vi "Exercise introduction.vi"(5 "Exercise Execution Mode":T1, 6 "Numero USP":dbl format="%#.13f", 7 "Exercise Number":T6, 8 "error in":errorcluster, 9 "Waveform In":waveform(dbl), 10 "Array":bool[](array[boolean]), 11 "Exercise Folder Path":path) -> (0 "error out":errorcluster, 1 "Waveform Out":waveform(dbl), 2 "Done":dbl, 3 "path":path)   [LabVIEW 2014]
uses:
  Ctls/t2q1.ctl
  Ctls/t2q2.ctl
  Ctls/ExerciseNumeration.ctl
  Ctls/ExerciseState.ctl
  Ctls/teval.ctl
  <vilib>/Utility/miscctls.llb/LVPointTypeDef.ctl
  Ctls/radiobutton010.ctl
panel:
  out "Exercise Tab":T2(tab)
  in  "Close 3":bool
  in  "TEVAL":T3 caption="Perguntas"
  in  "Close":bool
  in  "T2E1":T4 caption="Perguntas:"
  in  "Help? 2":bool
  out "Ex1 Graph Overview":waveform(dbl)(graph)
  in  "T2E2":T5={"Vmax (V)"=0.0, "Vmin (V)"=0.0, "Taxa de Aquisição (Hz)"=0.0, "Resolução (bits)"=0.0, "Amplificação (V/V)"=1.0, "V+(V)"=0.0, "V- (V)"=0.0, "LSB (V)"=0.0}
  in  "Close 2":bool
  in  "Help? 3":bool
  # "PSI3214\nLaboratório de Instrumentação Elétrica"
  # "Avaliação do Tutorial"
  # "Ao longo do tutorial foram utilizados materiais em PDF para referência do aluno, materiais em vídeo para acompanhamento mais dinâmico. Neste questionário serão avaliados alguns parâmetros quantitativos a fim de se melhorar a qualidade dos tutoriais fornecidos ao longo dos anos. É importante deixar claro que não será pedida nenhuma informação que possa identificar o aluno, de modo a preservar a privacidade de cada um."
  # "AA.1) Em relação ao Material Escrito disponibilizado em PDF, avalie:"
  # "Neste tutorial você foi apresentado a diversos conceitos sobre instrumentação elétrica e programação em LabVIEW. Em relação ao tamanho e à quantidade de conteúdo apresentado, você qualifica o tutorial como:"
  # "Pouco extenso\nPouco conteúdo"
  # "Pouco Extenso\nConteúdo adequado"
  # "Muito Extenso\nConteúdo adequado"
  # "Muito extenso\nPouco conteúdo"
  # "A realização dos tutoriais é importante para ter uma experiência completa do Laboratório de Instrumentação Elétrica. No entanto, é necessário um balanço entre as aulas teórias, experimentos e o exercícios em LabVIEW. Estime o tempo utilizado para a realização deste tutorial:"
  # "00h30-"
  # "00h30"
  # "01h00"
  # "01h30"
  # "02h00"
  # "02h30"
  # "03h00"
  # "03h30"
  # "04h00"
  # "04h00+"
  # "Este tutorial foi elaborado para ser realizado em conjunto com as disciplinas oferecidas no 4º semestre do curso de Engenharia Elétrica. Com relação aos conceitos abordados neste tutorial, indique, na sua opinião, que parcela do conteúdo foi apresentada adequadamente:"
  # "Nenhuma"
  # "Poucos"
  # "Maioria"
  # "Todos"
  # "Dada a quantidade de conceitos novos apresentados ao longo do tutorial, estime quantas leituras, em média, foram utilizadas para a compreensão de um tópico:"
  # "4 vezes +"
  # "3 vezes"
  # "2 vezes"
  # "1 vez"
  # "Apesar do tutorial apresentar novos conteúdos de programação, dentre outros conteúdos, sua proposta é de complementar as aulas teóricas e práticas de laboratório. Na sua opinião, estime como este tutorial auxiliou na compreensão dos assunto tratados na disciplina:"
  # "Dificultou\nmuito"
  # "Dificultou\npouco"
  # "Auxiliou\npouco"
  # "Auxiliou\nmuito"
  # "A instrumentação elétrica apresenta uma vasta gama de problemas de aquisição e processamento de dados. Para compreender melhor como aplicar os conceitos abordados na disciplina, neste tutorial foram apresentados alguns exemplos de problemas de instrumentação na forma de exercícios. Com relação aos problemas apresentados, indique como os exercícios propostos o auxiliaram em sua resolução:"
  # "Exercício não \najudou em nada"
  # "Exercício pouco \najudou na resolução"
  # "Exercício ajudou\nparcialmente na resolução"
  # "Exercício ajudou \nbastante na resolução"
  # "Diversos conceitos sobre programação em LabVIEW foram apresentados no tutorial. Tais ferramentas foram apresentadas com a intenção de ensiná-los como e quando utilizá-las. Estime o seu aprendizado a respeito de como utilizar tais ferramentas de programação e para qual finalidade aplicá-las:"
  # "Não sei como utilizar, \ne não sei sua finalidade"
  # "Sei como utilizar, mas \nnão sei sua finalidade"
  # "Não sei como utilizar, \nmas sei sua finalidade"
  # "Sei como utilizar, \ne sei sua finalidade"
  # "Indique como este tutorial colaborou na compreensão de assuntos abordados por outras disciplinas:"
  # "Nada"
  # "Pouco"
  # "Parcialmente"
  # "Muito"
  # "Indique seu conhecimento prévio a respeito do ambiente de programação em LabVIEW ante de realizar esse tutorial:"
  # "Não sabia o \nque era LabVIEW"
  # "Já tinha ouvido falar, mas \nnunca programei LabVIEW"
  # "Já programei LabVIEW\nalgumas vezes"
  # "Utilizo LabVIEW com\nalguma regularidade"
  # "Dada a resposta do item anterior, indique como classificaria seu aprendizado do conteúdo apresentado:"
  # "Todo o conteúdo\napresentado"
  # "Nada"
  # "Pouco"
  # "Parcialmente"
  # "PSI3214\nLaboratório de Instrumentação Elétrica"
  # "Exercício 2.1"
  # "Vimos ao longo do tutorial 2 que um sistema de aquisição possui como principal componente o ADC, Conversor Analógico Digital ou (Analog to Digital Converter). Para definição dos parâmentros que definem o ADC, tais como sua taxa de aquisição, fundo de escala e sua resolução, é necessário primeiro uma analise do sinal de entrada. Neste primeiro exercício iremos construir um projeto ingênuo de um ADC, desconsiderando algumas sutilezas presentes em sistemas de aquisição."
  # "Uma empresa de motores elétricos quer avaliar qual a precisão da construção de seus motores. Idealmente, os motores possuem rotação de 12000 RPM, contudo, defeitos na construção do eixo principal podem afetar a rotação. Como engenheiro de teste desta empresa à você foi encarregada a tarefa de construção de um sistema de aquisição para realizar tal avaliação. \n\nComo o sistema deve se móvel, você optou pela construção de um sensor de rotação ótico (figura ao lado). A cada rotação completa do eixo central do motor uma fita branca passa na frente do refletor IR, produzindo um pulso que será identificado pelo sistema de conversão AD."
  # "Utilize o sinal gerado no VI do exercicio para responder as perguntas abaixo:"
  # "Para fechar a tela do enunciado, pressione o botão \"Close Form\""
  # "A) Analise o sinal adquirido pelo ADC (em azul) e indique as características à seguir:"
  # "B) Sabe-se que o ADC utilizado para a aquisição inicial é de 10 bits e possui um LSB de aproximadamente 23,43mV. Indique o valor do fundo de escala:"
  # "C) Caso fosse requisitado que o ADC fosse sensível a variações do sinal de no mínimo 0,50mV. Indique os valores de,"
  # "PSI3214\nLaboratório de Instrumentação Elétrica"
  # "Exercício 2.2"
  # "Até o presente momento foi realizada uma apresentação ingênua do problema de aquisição de dados, na qual um conversor AD pode realizar aquisições de dados sem a introdução de erros ou ruídos no sinal qualquer que seja sua tensão de alimentação. Contudo, como discutido no tutorial, não é recomendado que a tensão de alimentação de um conversor seja pequena. Dados os circuitos integrados disponíveis no mercado, tensões de 5V são algumas das mais comuns para aplicações ordinárias."
  # "Como todos os sistemas que operam no mundo real, sempre serão introduzidos erros no sinal. É também trabalho do engenheiro identificar essas fontes de erros e buscar minimizar seus efeitos na análise final. Para o caso específico dos Conversores AD, são introduzidos erros proporcionais àqueles presentes na alimentação do ADC, bem como erros introduzidos por indutâncias e capacitâncias parasitárias. Quando  a tensão de alimentação é muito baixa, a proporção entre os erros introduzidos e o sinal de interesse aumenta, algo indesejado, especialmente para o caso de sinais de baixa amplitude. Caso utilizemos um conversor AD em conjunto com um amplificador, podemos aumentar os níveis do sinal, efetivamente diminuindo a proporção entre erro introduzido e o sinal, como mostra a figura abaixo."
  # "Um dos temas em Engenharia que tem maior adesão da mídia é o de Cidades Inteligentes e a sua construção por meio de sistemas embarcados, capazes de realizar aquisição de dados, processamento e a comunicação desses dados para outros sistemas. Contudo, a ideia de se colocar sensores em uma cidade afim de se monitorar condições como tráfego, níveis de ruído, dentre outros parâmetros não é uma ideia nova. No final dos anos 90 nos EUA, com o aumento dos índices de criminalidade em cidades grandes foram implementados os primeiros projetos de identificação de dispáro de tiros em algumas das principais vias das maiores cidades. Apesar de a classificassão do sinal como sendo de uma arma de fogo ou de uma batida de carro ser um assunto complexo, o sistema de aquisição de dados é, de certo modo, simples. \n    Neste exercício vamos utilizar o diagrama de blocos descrito anteriormente como a topologia de nosso projeto. Como definido acima, iremos fazer uso de um aplificador antes do processo de conversão AD.\n    Utilize o sinal gerado no VI principal para realizar as medições pertinentes:"
  # "A) Descreva o sinal a ser adquirido (em vermelho), indicando:"
  # "- Níveis de Tensão Globais Máximo e Mínimo:"
  # "Na modelagem sonora de uma arma de fogo, sugere-se que para maioria das armas comercializadas estamos interessados em sinais de até 2kHz, sendo assim:"
  # "B) Dado que 20x a Frequência de Nyquist é um valor utilizado em engenharia como mais do que \nadequado para o processo de aquisição de dados, selecione qual a taxa de aquisição mínima mais \naceitável para o conversor AD:"
  # "C) Dado que a tensão de fundo de escala do conversor é de 10V e que desejamos utilzar ao máximo os endereços binários com informação util: Qual a amplificação que deverá ser dada ao sinal (em vermelho)? Dado que o sinal é simétrico, quais as tensões de alimentação do conversor AD para que tenha a tensão de fundo de escala necessária?"
  # "Como etapa final do projeto, queremos que quaisquer variações de sinal menores ou da ordem de 1mV sejam detectadas pelo conversor, deste modo:"
  # "D) Selecione qual a resolução mínima para que essa especificação seja cumprida e qual o LSB resultante desta configuração, considerando a tensão do fundo de escala dada no item C."
  # "Para fechar a tela do enunciado, pressione o botão \"Close Form\""
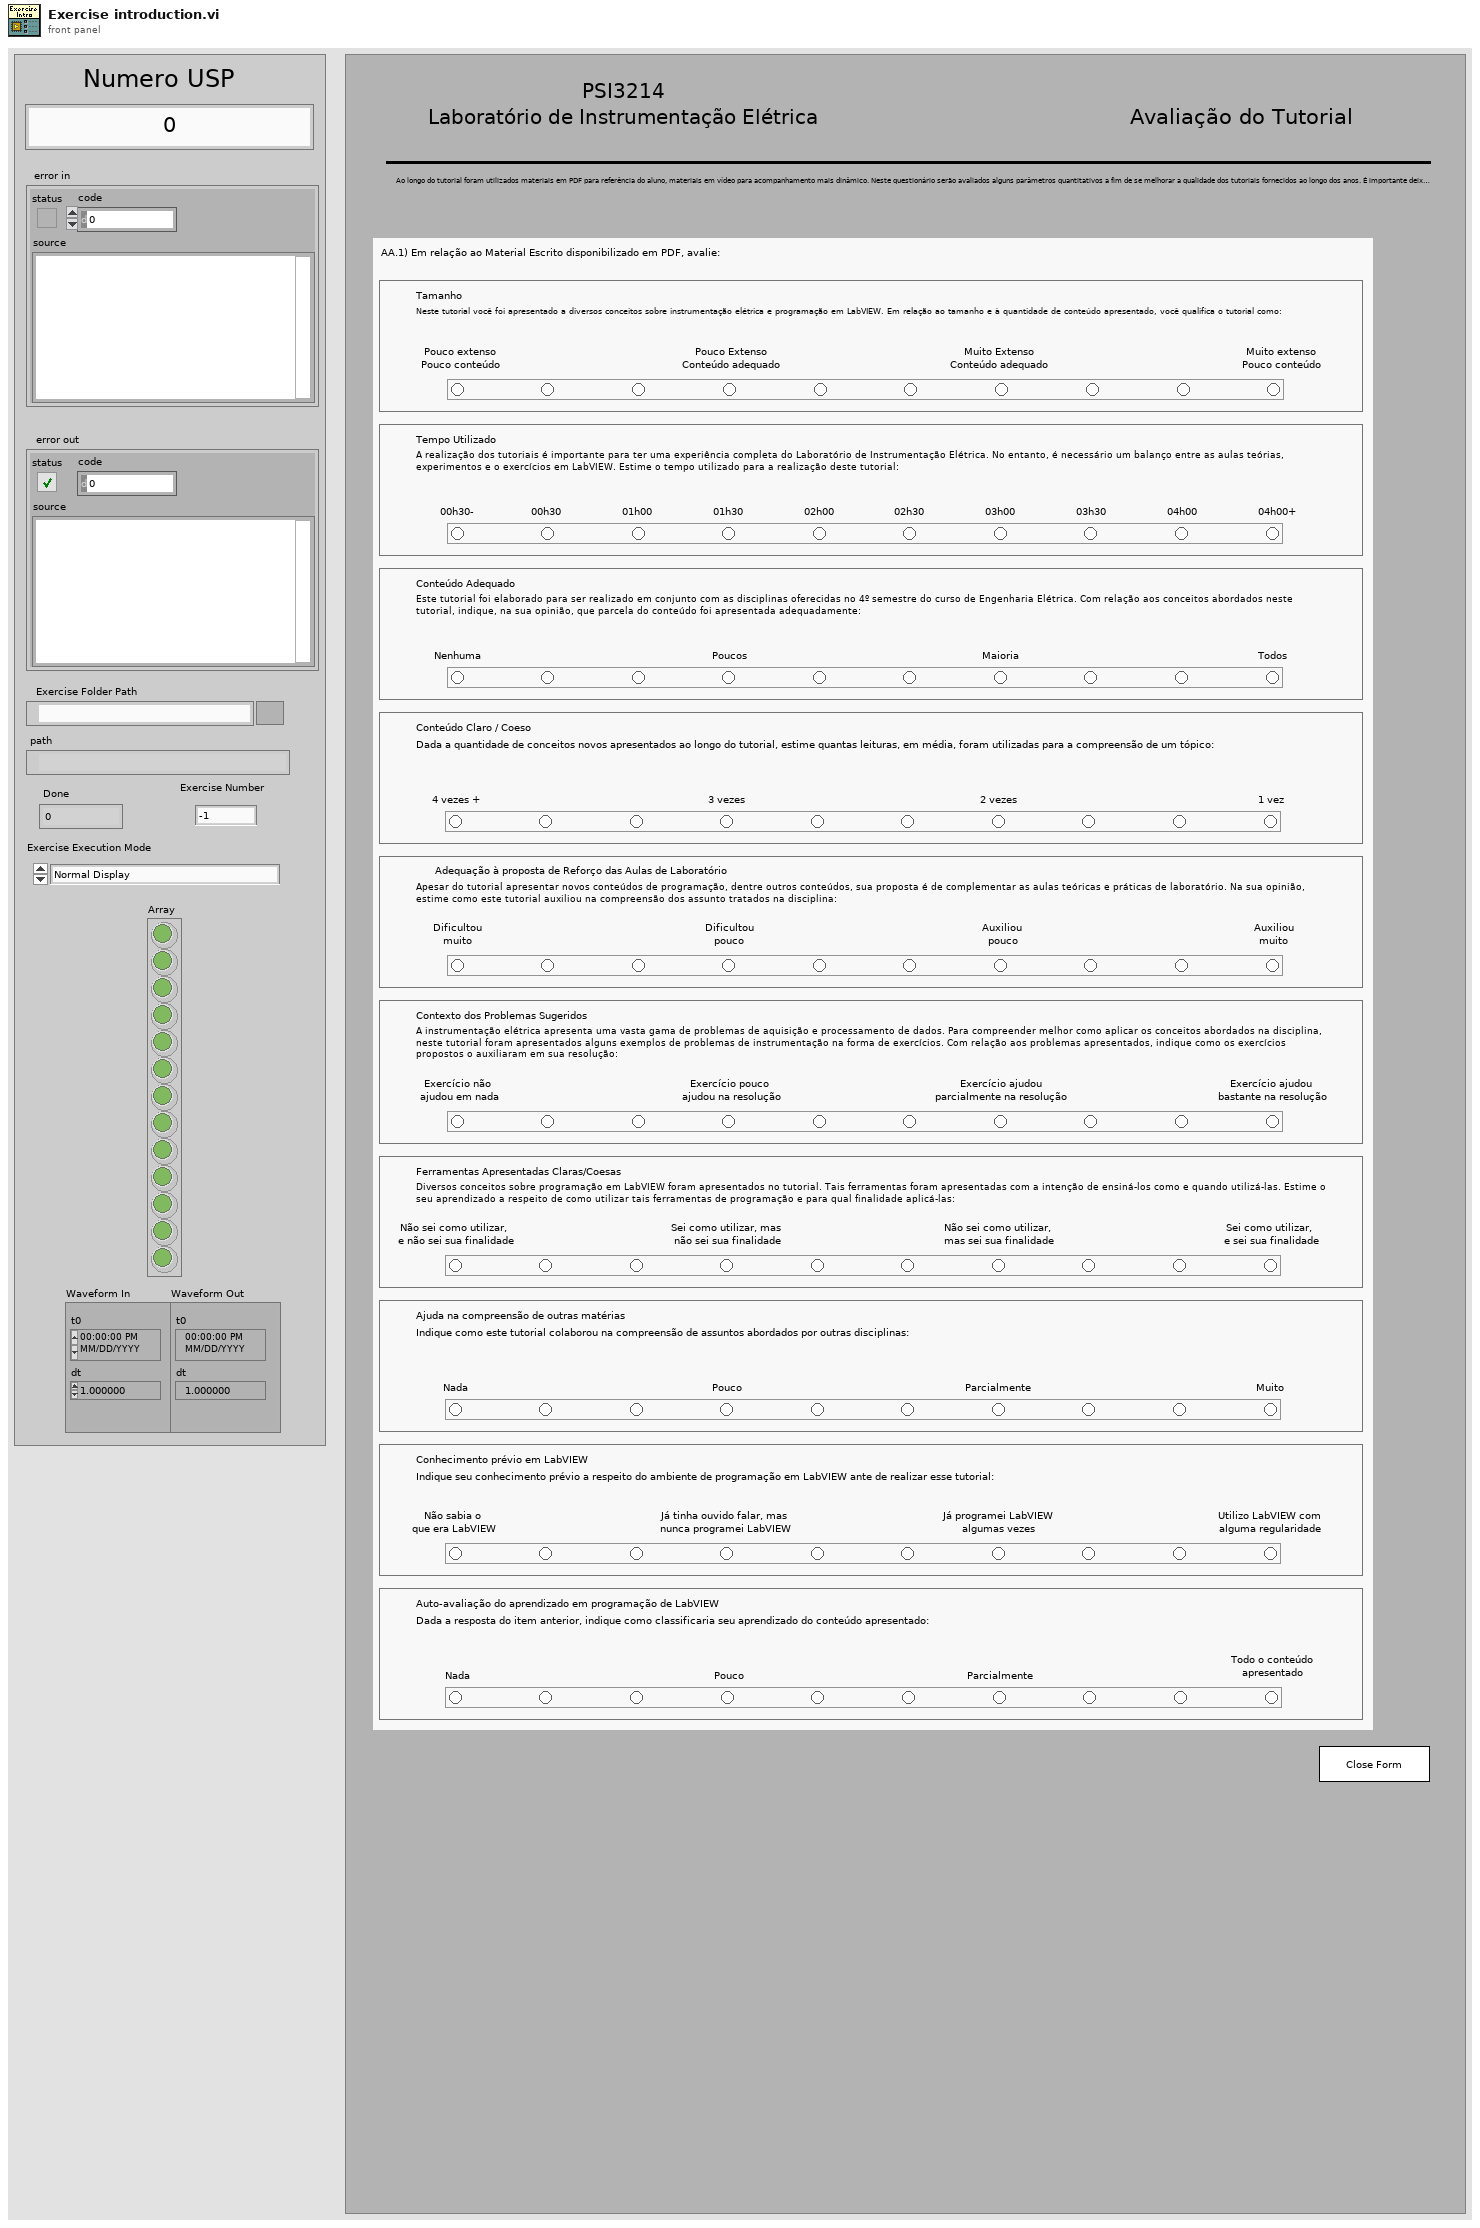
[diagram p1: front panel]
types:
  T1 = typedef "ExerciseState.ctl" = enum16{"Normal Display", "Answer Highligh"}
  T2 = enum32{"Tutorial Evaluation", "Exercicio 1", "Exercicio 2", "Exercício 3", "Exercício 4", "Exercício 5"}
  T3 = typedef "teval.ctl" = cluster{"Tamanho":enum32{"No Selection", "2", "1", "3", "4", "5", "6", "7", "8", "9", "10"}, "Tempo Utilizado":enum32{"No Selection", "2", "1", "3", "4", "5", "6", "7", "8", "9", "10"}, "Conteúdo Adequado":enum32{"No Selection", "2", "1", "3", "4", "5", "6", "7", "8", "9", "10"}, "Conteúdo Claro / Coeso":enum32{"No Selection", "2", "1", "3", "4", "5", "6", "7", "8", "9", "10"}, "Adequação à proposta de Reforço das Aulas de Laboratório e de Ensino de LabVIEW":enum32{"No Selection", "2", "1", "3", "4", "5", "6", "7", "8", "9", "10"}, "Contexto dos Problemas Sugeridos":enum32{"No Selection", "2", "1", "3", "4", "5", "6", "7", "8", "9", "10"}, "Contexto das Ferramentas Apresentadas":enum32{"No Selection", "2", "1", "3", "4", "5", "6", "7", "8", "9", "10"}, "Ajuda na compreensão de outras matérias":enum32{"No Selection", "2", "1", "3", "4", "5", "6", "7", "8", "9", "10"}, "compreensão de programação em LabVIEW":enum32{"No Selection", "2", "1", "3", "4", "5", "6", "7", "8", "9", "10"}, "compreensão da teoria apresentada":enum32{"No Selection", "2", "1", "3", "4", "5", "6", "7", "8", "9", "10"}}
  T4 = typedef "t2q1.ctl" = cluster{"Vmax (V)":dbl, "Vmin (V)":dbl, "Período (s)":dbl, "Fundo de Escala (V)":dbl, "Frequência de \nAmostragem \n[Hz]":dbl, "LSB (V)":dbl, "Resolução (bits)":dbl}
  T5 = typedef "t2q2.ctl" = cluster{"Vmax (V)":dbl, "Vmin (V)":dbl, "Taxa de Aquisição (Hz)":dbl, "Resolução (bits)":dbl, "Amplificação (V/V)":dbl, "V+(V)":dbl, "V- (V)":dbl, "LSB (V)":dbl}
  T6 = typedef "ExerciseNumeration.ctl" = enum16{"-1", "0", "1", "2", "3", "4", "5", "6", "7", "8", "9", "10"}
  T7 = typedef "LVPointTypeDef.ctl" = cluster{"Horizontal":i16, "Vertical":i16}
  T8 = enum16{"Always On", "Always Off", "Off While Running"}
  T9 = enum16{"open", "replace", "create", "open or create", "replace or create", "replace or create with confirmation"}
  T10 = typedef "radiobutton010.ctl" = enum32{"No Selection", "2", "1", "3", "4", "5", "6", "7", "8", "9", "10"}
  T11 = enum32{"No Selection", "2", "1", "3", "4", "5", "6", "7", "8", "9", "10"}
  T12 = enum32{"No Selection", "2", "1", "3", "4", "5", "6", "7", "8", "9", "10"}[]
  T13 = typedef "imagedata.ctl" = cluster{"image type":i32, "image depth":i32, "image":u8[], "mask":u8[], "colors":u32[], "Rectangle":cluster{"left":i16, "top":i16, "right":i16, "bottom":i16}}
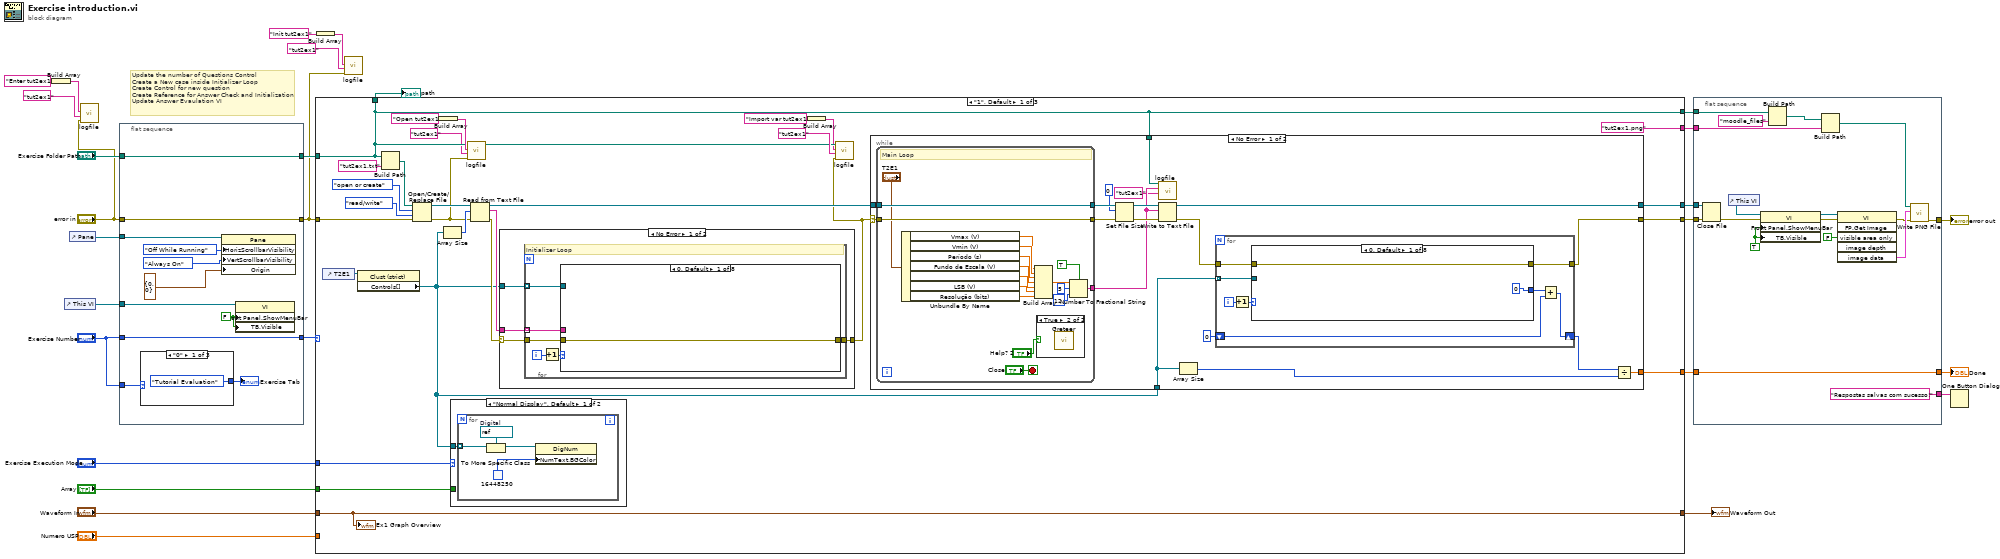
[diagram p0: block diagram]
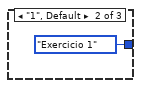
[diagram p2: hidden frame]
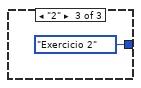
[diagram p3: hidden frame]
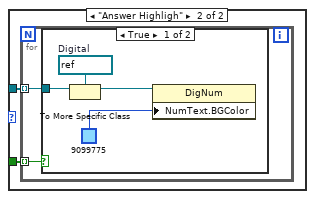
[diagram p4: hidden frame]
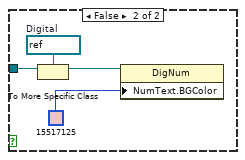
[diagram p5: hidden frame]
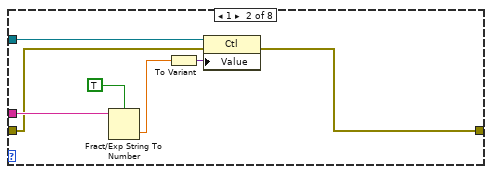
[diagram p6: hidden frame]
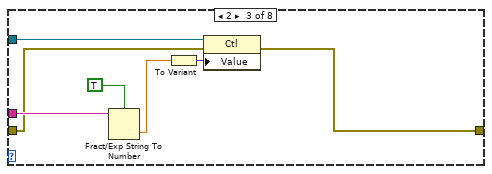
[diagram p7: hidden frame]
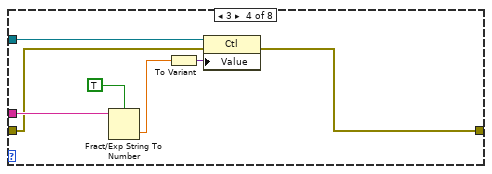
[diagram p8: hidden frame]
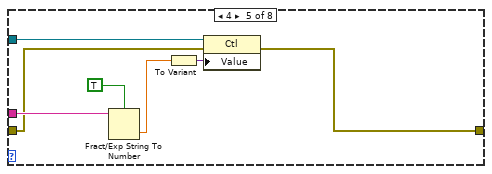
[diagram p9: hidden frame]
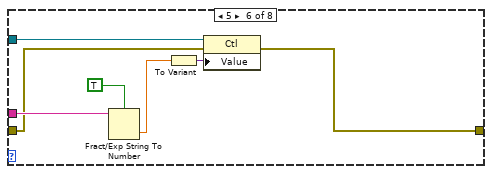
[diagram p10: hidden frame]
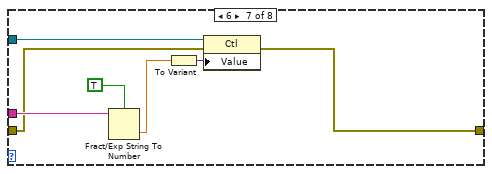
[diagram p11: hidden frame]
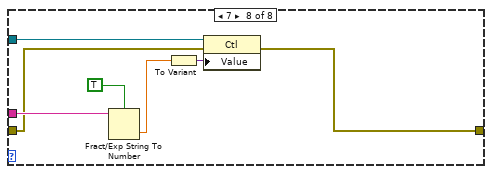
[diagram p12: hidden frame]
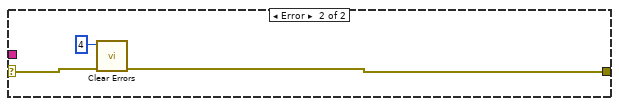
[diagram p13: hidden frame]
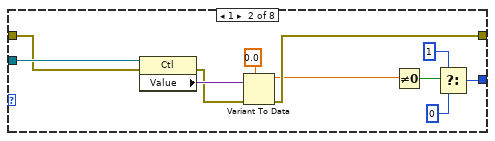
[diagram p14: hidden frame]
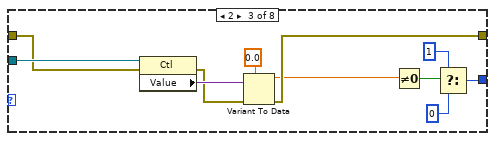
[diagram p15: hidden frame]
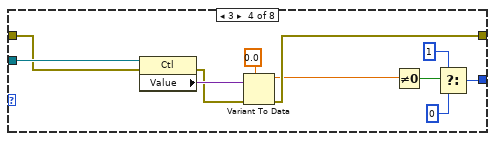
[diagram p16: hidden frame]
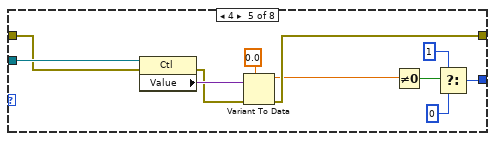
[diagram p17: hidden frame]
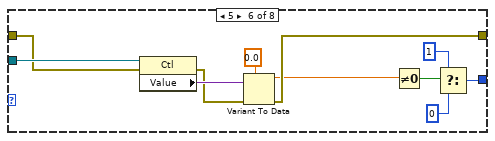
[diagram p18: hidden frame]
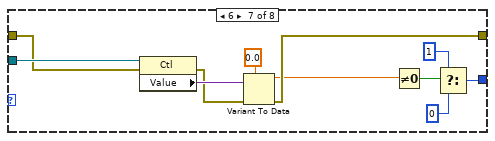
[diagram p19: hidden frame]
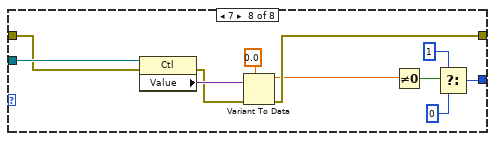
[diagram p20: hidden frame]
diagram:
  # "Update the number of Questions Control\nCreate a New case inside Initializer Loop\nCreate Control for new question\nCreate Reference for Answer Check and Initialization\nUpdate Answer Evaulation VI"
  n1 = Build Array("Enter tut2ex1") -> (w7:string[])
  n2 = control-ref of="This VI"() -> (w26:refnum<vi>)
  n3 = control-ref of="Pane"() -> (w17:refnum<vi>)
  n4 = call "logfile.vi"("Error In"="error in", "Locale"="tut2ex1", "Text In"=w7) -> ()  [unwired: 7 in, 2 out]
  n5 = flat-sequence {
    tunnel: "Exercise Number" -> [w39]
    tunnel: w17 -> [w38]
    tunnel: w26 -> [w37]
    tunnel: "error in" -> [w33]
    tunnel: [w33] -> w2
    tunnel: "Exercise Folder Path" -> [w36]
    tunnel: [w36] -> w24
    tunnel: "Exercise Number" -> [w32]
    tunnel: [w32] -> w22
    frame #0 {
      w35 = FALSE ("Front Panel Window:Show Menu Bar")
      n6 = case shown="\"0\"" w39 {
        tunnel: [T2."Tutorial Evaluation" ("Exercise Tab") T2."Exercicio 1" ("Exercise Tab") T2."Exercicio 2" ("Exercise Tab")] -> w30
        frame "0" {
        }
        frame "1", Default {
        }
        frame "2" {
        }
      }
      "Exercise Tab" <- w30
      n7 = property class="Pane"(reference=w38, "HorizScrollbarVisibility"=T8."Off While Running" ("Horizontal Scrollbar Visibility"), "VertScrollbarVisibility"=T8."Always On" ("Vertical Scrollbar Visibility"), "Origin"=T7 {"Horizontal"=0, "Vertical"=0}) -> ()  [unwired: 1 in, 2 out]
      n8 = property class="VI"(reference=w37, "Front Panel.ShowMenuBar"=w35, "TB.Visible"=w35) -> ()  [unwired: 1 in, 2 out]
    }
  }
  n9 = case shown="\"1\", Default" w22 {
    tunnel: w24 -> [w50 w278 w514]
    tunnel: w2 -> [w69 w296 w531]
    tunnel: [w64 w290 w525] -> w28
    tunnel: [w63 w289 w524] -> w27
    tunnel: [w60 w285 w520] -> w19
    tunnel: [w50 w278 w514] -> w18
    tunnel: "Array" -> [w55 w280 _]
    tunnel: "Exercise Execution Mode" -> [w56 w281 _]
    tunnel: "Waveform In" -> [w54 w282 w517]
    tunnel: [w54 w282 w517] -> w13
    tunnel: "Numero USP" -> [_ _ _]
    tunnel: [w50 w278 w514] -> w11
    tunnel: ["tut2ex1.png" ("name or relative path") "tut2ex2.png" ("name or relative path") "tut2eval.png" ("name or relative path")] -> w9
    frame "1", Default {
      n10 = control-ref of="T2E1"() -> (w58:refnum<vi>)
      n11 = property class="Clust (strict)"(reference=w58) -> ("Controls[]"=w57:refnum<vi>[])  [unwired: 1 in, 2 out]
      n12 = Build Path(base path=w50, name or relative path="tut2ex1.txt") -> (appended path=w70:path)
      n13 = Open/Create/Replace File(file path (use dialog)=w70, error in=w69, operation (0:open)=T9."open or create", access (0:read/write)=enum16{"read/write", "read-only", "write-only"}."read/write") -> (refnum out=w66:refnum<file>, error out=w48:errorcluster)  [unwired: 2 in, 1 out]
      n14 = Build Array("Open tut2ex1") -> (w51:string[])
      n15 = Array Size(array=w57) -> (size(s)=w59:i32)
      n16 = case shown="\"Normal Display\", Default" w56 {
        tunnel: w57 -> [w72 w78]
        tunnel: w55 -> [_ w77]
        frame "Normal Display", Default {
          n17 = for {
            tunnel: w72 -> [w76] mode=indexing
            w74 = refnum<vi> refnum  # Digital
            n18 = To More Specific Class(target class=w74, reference=w76) -> (specific class reference=w75:refnum<vi>)  [unwired: 1 in, 1 out]
            n19 = property class="DigNum"(reference=w75, "NumText.BGColor"=u32 16448250) -> ()  [unwired: 1 in, 2 out]
          }
        }
        frame "Answer Highligh" {
          n20 = for {
            tunnel: w78 -> [w80] mode=indexing
            tunnel: w77 -> [w79] mode=indexing
            n21 = case shown="True" w79 {
              tunnel: w80 -> [w83 w88]
              frame True {
                w81 = refnum<vi> refnum  # Digital
                n22 = To More Specific Class(target class=w81, reference=w83) -> (specific class reference=w82:refnum<vi>)  [unwired: 1 in, 1 out]
                n23 = property class="DigNum"(reference=w82, "NumText.BGColor"=u32 9099775) -> ()  [unwired: 1 in, 2 out]
              }
              frame False {
                w86 = refnum<vi> refnum  # Digital
                n24 = To More Specific Class(target class=w86, reference=w88) -> (specific class reference=w87:refnum<vi>)  [unwired: 1 in, 1 out]
                n25 = property class="DigNum"(reference=w87, "NumText.BGColor"=u32 15517125) -> ()  [unwired: 1 in, 2 out]
              }
            }
          }
        }
      }
      n26 = call "logfile.vi"("Error In"=w48, "Locale"="tut2ex1", "Text In"=w51, "Path In"=w50) -> ("Path Out"=w46:path)  [unwired: 6 in, 1 out]
      n27 = Read from Text File(file (use dialog)=w66, count=w59, error in=w48) -> (refnum out=w65:refnum<file>, text=w61:string[], error out=w62:errorcluster)  [unwired: 1 in, 1 out]
      n28 = case shown="No Error" w62 {
        selector: w62 -> [w91 w151]
        tunnel: w61 -> [w92 _]
        tunnel: [w90 w150] -> w43
        tunnel: w57 -> [w89 _]
        frame No Error {
          n29 = for {
            tunnel: w92 -> [w98] mode=indexing
            tunnel: [w95] -> w90
            tunnel: w91 -> [w94]
            tunnel: w89 -> [w93] mode=indexing
            i -> [w96]
            # "Initializer Loop"
            n30 = Increment(x=w96) -> (x+1=w97:i32)
            n31 = case shown="0, Default" w97 {
              tunnel: w98 -> [_ w104 w111 w118 w125 w132 w139 w146]
              tunnel: [w99 w106 w113 w120 w127 w134 w141 w148] -> w95
              tunnel: w94 -> [w99 w100 w107 w114 w121 w128 w135 w142]
              tunnel: w93 -> [_ w105 w112 w119 w126 w133 w140 w147]
              frame 0, Default {
              }
              frame 1 {
                n32 = Fract/Exp String To Number(use system decimal point (T)=TRUE, string=w104) -> (number=w102:dbl)  [unwired: 2 in, 1 out]
                n33 = To Variant(anything=w102) -> (Variant=w103:variant)
                n34 = property class="Ctl"(reference=w105, error in=w100, "Value"=w103) -> (error out=w106:errorcluster)  [unwired: 1 out]
              }
              frame 2 {
                n35 = Fract/Exp String To Number(use system decimal point (T)=TRUE, string=w111) -> (number=w109:dbl)  [unwired: 2 in, 1 out]
                n36 = To Variant(anything=w109) -> (Variant=w110:variant)
                n37 = property class="Ctl"(reference=w112, error in=w107, "Value"=w110) -> (error out=w113:errorcluster)  [unwired: 1 out]
              }
              frame 3 {
                n38 = Fract/Exp String To Number(use system decimal point (T)=TRUE, string=w118) -> (number=w116:dbl)  [unwired: 2 in, 1 out]
                n39 = To Variant(anything=w116) -> (Variant=w117:variant)
                n40 = property class="Ctl"(reference=w119, error in=w114, "Value"=w117) -> (error out=w120:errorcluster)  [unwired: 1 out]
              }
              frame 4 {
                n41 = Fract/Exp String To Number(use system decimal point (T)=TRUE, string=w125) -> (number=w123:dbl)  [unwired: 2 in, 1 out]
                n42 = To Variant(anything=w123) -> (Variant=w124:variant)
                n43 = property class="Ctl"(reference=w126, error in=w121, "Value"=w124) -> (error out=w127:errorcluster)  [unwired: 1 out]
              }
              frame 5 {
                n44 = Fract/Exp String To Number(use system decimal point (T)=TRUE, string=w132) -> (number=w130:dbl)  [unwired: 2 in, 1 out]
                n45 = To Variant(anything=w130) -> (Variant=w131:variant)
                n46 = property class="Ctl"(reference=w133, error in=w128, "Value"=w131) -> (error out=w134:errorcluster)  [unwired: 1 out]
              }
              frame 6 {
                n47 = Fract/Exp String To Number(use system decimal point (T)=TRUE, string=w139) -> (number=w137:dbl)  [unwired: 2 in, 1 out]
                n48 = To Variant(anything=w137) -> (Variant=w138:variant)
                n49 = property class="Ctl"(reference=w140, error in=w135, "Value"=w138) -> (error out=w141:errorcluster)  [unwired: 1 out]
              }
              frame 7 {
                n50 = Fract/Exp String To Number(use system decimal point (T)=TRUE, string=w146) -> (number=w144:dbl)  [unwired: 2 in, 1 out]
                n51 = To Variant(anything=w144) -> (Variant=w145:variant)
                n52 = property class="Ctl"(reference=w147, error in=w142, "Value"=w145) -> (error out=w148:errorcluster)  [unwired: 1 out]
              }
            }
          }
        }
        frame Error {
          n53 = call <vilib>:"Clear Errors.vi"("error in (no error)"=w151, "specific error code to clear (0: all)"=4) -> ("error out"=w150:errorcluster)  [unwired: 4 in, 1 out]
        }
      }
      n54 = Build Array("Import var tut2ex1") -> (w45:string[])
      n55 = call "logfile.vi"("Error In"=w43, "Locale"="tut2ex1", "Text In"=w45, "Path In"=w46) -> ()  [unwired: 6 in, 2 out]
      n56 = case shown="No Error" w43 {
        selector: w43 -> [w168 w275]
        tunnel: w65 -> [w169 w276]
        tunnel: [w156 w275] -> w64
        tunnel: [w167 w276] -> w63
        tunnel: [w160 -1.0] -> w60
        tunnel: w57 -> [w159 _]
        tunnel: w50 -> [w152 _]
        frame No Error {
          n57 = while {
            tunnel: w169 -> [w272]
            tunnel: w168 -> [w271]
            tunnel: [w272] -> w164
            tunnel: [w271] -> w166
            tunnel: [w265] -> w154
            stop <- "Close" stop-if-true
            # "Main Loop"
            n58 = Unbundle By Name("T2E1") -> ("Vmax (V)"=w259:dbl, "Vmin (V)"=w260:dbl, "Período (s)"=w270:dbl, "Fundo de Escala (V)"=w269:dbl, "Frequência de \nAmostragem \n[Hz]"=w268:dbl, "LSB (V)"=w267:dbl, "Resolução (bits)"=w266:dbl)
            n59 = Build Array(w259, w260, w270, w269, w268, w267, w266) -> (w264:dbl[])
            n60 = case shown="True" "Help? 2" {
              frame False {
              }
              frame True {
                n61 = call "Greteer.vi"() -> ()  [unwired: 10 in, 2 out]
              }
            }
            n62 = Number To Fractional String(use system decimal point (T)=TRUE, number=w264, width (-)=i16 5, precision (6)=i16 12) -> (F-format string=w265:string[])
          }
          n63 = Set File Size(4:w166, 6:i64 0 ("size (in bytes)"), 7:w164) -> (0:w165:errorcluster, 3:w163:refnum<file>)
          n64 = Write to Text File(file (use dialog)=w163, text=w154, error in=w165) -> (refnum out=w167:refnum<file>, error out=w157:errorcluster)  [unwired: 1 in, 1 out]
          n65 = call "logfile.vi"("Locale"="tut2ex1" ("from"), "Text In"=w154, "Path In"=w152) -> ()  [unwired: 7 in, 2 out]
          n66 = Array Size(array=w159) -> (size(s)=w158:i32)
          n67 = for {
            shift-right: [w174] -> w161
            shift-left: 0 -> [w173]
            tunnel: w159 -> [w172] mode=indexing
            tunnel: w157 -> [w171]
            tunnel: [w170] -> w156
            i -> [w176]
            n68 = Increment(x=w176) -> (x+1=w177:i32)
            n69 = case shown="0, Default" w177 {
              tunnel: [0 ("f") w188 w199 w210 w221 w232 w243 w254] -> w175
              tunnel: w172 -> [_ w185 w196 w207 w218 w229 w240 w251]
              tunnel: w171 -> [w178 w184 w195 w206 w217 w228 w239 w250]
              tunnel: [w178 w182 w193 w204 w215 w226 w237 w248] -> w170
              frame 0, Default {
              }
              frame 1 {
                n70 = property class="Ctl"(reference=w185, error in=w184) -> (error out=w183:errorcluster, "Value"=w186:variant)  [unwired: 1 out]
                n71 = Variant To Data(error in=w183, type=0.0 ("y"), Variant=w186) -> (data=w180:dbl, error out=w182:errorcluster)
                n72 = Not Equal To 0?(x=w180) -> (x != 0?=w181:bool)
                n73 = Select(t=1, s=w181, f=0) -> (s? t:f=w188:i32)
              }
              frame 2 {
                n74 = property class="Ctl"(reference=w196, error in=w195) -> (error out=w194:errorcluster, "Value"=w197:variant)  [unwired: 1 out]
                n75 = Variant To Data(error in=w194, type=0.0 ("y"), Variant=w197) -> (data=w191:dbl, error out=w193:errorcluster)
                n76 = Not Equal To 0?(x=w191) -> (x != 0?=w192:bool)
                n77 = Select(t=1, s=w192, f=0) -> (s? t:f=w199:i32)
              }
              frame 3 {
                n78 = property class="Ctl"(reference=w207, error in=w206) -> (error out=w205:errorcluster, "Value"=w208:variant)  [unwired: 1 out]
                n79 = Variant To Data(error in=w205, type=0.0 ("y"), Variant=w208) -> (data=w202:dbl, error out=w204:errorcluster)
                n80 = Not Equal To 0?(x=w202) -> (x != 0?=w203:bool)
                n81 = Select(t=1, s=w203, f=0) -> (s? t:f=w210:i32)
              }
              frame 4 {
                n82 = property class="Ctl"(reference=w218, error in=w217) -> (error out=w216:errorcluster, "Value"=w219:variant)  [unwired: 1 out]
                n83 = Variant To Data(error in=w216, type=0.0 ("y"), Variant=w219) -> (data=w213:dbl, error out=w215:errorcluster)
                n84 = Not Equal To 0?(x=w213) -> (x != 0?=w214:bool)
                n85 = Select(t=1, s=w214, f=0) -> (s? t:f=w221:i32)
              }
              frame 5 {
                n86 = property class="Ctl"(reference=w229, error in=w228) -> (error out=w227:errorcluster, "Value"=w230:variant)  [unwired: 1 out]
                n87 = Variant To Data(error in=w227, type=0.0 ("y"), Variant=w230) -> (data=w224:dbl, error out=w226:errorcluster)
                n88 = Not Equal To 0?(x=w224) -> (x != 0?=w225:bool)
                n89 = Select(t=1, s=w225, f=0) -> (s? t:f=w232:i32)
              }
              frame 6 {
                n90 = property class="Ctl"(reference=w240, error in=w239) -> (error out=w238:errorcluster, "Value"=w241:variant)  [unwired: 1 out]
                n91 = Variant To Data(error in=w238, type=0.0 ("y"), Variant=w241) -> (data=w235:dbl, error out=w237:errorcluster)
                n92 = Not Equal To 0?(x=w235) -> (x != 0?=w236:bool)
                n93 = Select(t=1, s=w236, f=0) -> (s? t:f=w243:i32)
              }
              frame 7 {
                n94 = property class="Ctl"(reference=w251, error in=w250) -> (error out=w249:errorcluster, "Value"=w252:variant)  [unwired: 1 out]
                n95 = Variant To Data(error in=w249, type=0.0 ("y"), Variant=w252) -> (data=w246:dbl, error out=w248:errorcluster)
                n96 = Not Equal To 0?(x=w246) -> (x != 0?=w247:bool)
                n97 = Select(t=1, s=w247, f=0) -> (s? t:f=w254:i32)
              }
            }
            n98 = Add(x=w175, y=w173) -> (x+y=w174:i32)
          }
          n99 = Divide(x=w161, y=w158) -> (x/y=w160:dbl)
        }
        frame Error {
        }
      }
      "Ex1 Graph Overview" <- w54
    }
    frame "2" {
      n100 = control-ref of="T2E2"() -> (w283:refnum<vi>)
      n101 = property class="Clust (strict)"(reference=w283) -> ("Controls[]"=w279:refnum<vi>[])  [unwired: 1 in, 2 out]
      n102 = Build Path(base path=w278, name or relative path="tut2ex2.txt") -> (appended path=w297:path)
      n103 = Open/Create/Replace File(file path (use dialog)=w297, error in=w296, operation (0:open)=T9."open or create", access (0:read/write)=enum16{"read/write", "read-only", "write-only"}."read/write") -> (refnum out=w293:refnum<file>, error out=w292:errorcluster)  [unwired: 2 in, 1 out]
      n104 = case shown="\"Answer Highligh\"" w281 {
        tunnel: w279 -> [w299 w305]
        tunnel: w280 -> [_ w304]
        frame "Normal Display", Default {
          n105 = for {
            tunnel: w299 -> [w303] mode=indexing
            w301 = refnum<vi> refnum  # Digital
            n106 = To More Specific Class(target class=w301, reference=w303) -> (specific class reference=w302:refnum<vi>)  [unwired: 1 in, 1 out]
            n107 = property class="DigNum"(reference=w302, "NumText.BGColor"=u32 16448250) -> ()  [unwired: 1 in, 2 out]
          }
        }
        frame "Answer Highligh" {
          n108 = for {
            tunnel: w305 -> [w307] mode=indexing
            tunnel: w304 -> [w306] mode=indexing
            n109 = case shown="True" w306 {
              tunnel: w307 -> [w310 w315]
              frame True {
                w308 = refnum<vi> refnum  # Digital
                n110 = To More Specific Class(target class=w308, reference=w310) -> (specific class reference=w309:refnum<vi>)  [unwired: 1 in, 1 out]
                n111 = property class="DigNum"(reference=w309, "NumText.BGColor"=u32 9099775) -> ()  [unwired: 1 in, 2 out]
              }
              frame False {
                w313 = refnum<vi> refnum  # Digital
                n112 = To More Specific Class(target class=w313, reference=w315) -> (specific class reference=w314:refnum<vi>)  [unwired: 1 in, 1 out]
                n113 = property class="DigNum"(reference=w314, "NumText.BGColor"=u32 15517125) -> ()  [unwired: 1 in, 2 out]
              }
            }
          }
        }
      }
      n114 = Array Size(array=w279) -> (size(s)=w284:i32)
      n115 = Read from Text File(file (use dialog)=w293, count=w284, error in=w292) -> (refnum out=w291:refnum<file>, text=w287:string[], error out=w288:errorcluster)  [unwired: 1 in, 1 out]
      n116 = case shown="No Error" w288 {
        selector: w288 -> [w318 w377]
        tunnel: w287 -> [w319 _]
        tunnel: [w317 w376] -> w286
        tunnel: w279 -> [w316 _]
        frame No Error {
          n117 = for {
            tunnel: w319 -> [w322] mode=indexing
            tunnel: [w320] -> w317
            tunnel: w318 -> [w323]
            tunnel: w316 -> [w321] mode=indexing
            i -> [w325]
            # "Initializer Loop"
            n118 = Increment(x=w325) -> (x+1=w324:i32)
            n119 = case shown="2" w324 {
              tunnel: w322 -> [_ w330 w336 w342 w348 w354 w360 w366 w372]
              tunnel: [errorcluster {"status"=FALSE, "code"=0, "source"=""} ("error out") w332 w338 w344 w350 w356 w362 w368 w374] -> w320
              tunnel: w321 -> [_ w331 w337 w343 w349 w355 w361 w367 w373]
              tunnel: w323 -> [_ _ _ _ _ _ _ _ _]
              frame 0, Default {
              }
              frame 1 {
                n120 = Fract/Exp String To Number(use system decimal point (T)=TRUE, string=w330) -> (number=w328:dbl)  [unwired: 2 in, 1 out]
                n121 = To Variant(anything=w328) -> (Variant=w329:variant)
                n122 = property class="Ctl"(reference=w331, "Value"=w329) -> (error out=w332:errorcluster)  [unwired: 1 in, 1 out]
              }
              frame 2 {
                n123 = Fract/Exp String To Number(use system decimal point (T)=TRUE, string=w336) -> (number=w334:dbl)  [unwired: 2 in, 1 out]
                n124 = To Variant(anything=w334) -> (Variant=w335:variant)
                n125 = property class="Ctl"(reference=w337, "Value"=w335) -> (error out=w338:errorcluster)  [unwired: 1 in, 1 out]
              }
              frame 3 {
                n126 = Fract/Exp String To Number(use system decimal point (T)=TRUE, string=w342) -> (number=w340:dbl)  [unwired: 2 in, 1 out]
                n127 = To Variant(anything=w340) -> (Variant=w341:variant)
                n128 = property class="Ctl"(reference=w343, "Value"=w341) -> (error out=w344:errorcluster)  [unwired: 1 in, 1 out]
              }
              frame 4 {
                n129 = Fract/Exp String To Number(use system decimal point (T)=TRUE, string=w348) -> (number=w346:dbl)  [unwired: 2 in, 1 out]
                n130 = To Variant(anything=w346) -> (Variant=w347:variant)
                n131 = property class="Ctl"(reference=w349, "Value"=w347) -> (error out=w350:errorcluster)  [unwired: 1 in, 1 out]
              }
              frame 5 {
                n132 = Fract/Exp String To Number(use system decimal point (T)=TRUE, string=w354) -> (number=w352:dbl)  [unwired: 2 in, 1 out]
                n133 = To Variant(anything=w352) -> (Variant=w353:variant)
                n134 = property class="Ctl"(reference=w355, "Value"=w353) -> (error out=w356:errorcluster)  [unwired: 1 in, 1 out]
              }
              frame 6 {
                n135 = Fract/Exp String To Number(use system decimal point (T)=TRUE, string=w360) -> (number=w358:dbl)  [unwired: 2 in, 1 out]
                n136 = To Variant(anything=w358) -> (Variant=w359:variant)
                n137 = property class="Ctl"(reference=w361, "Value"=w359) -> (error out=w362:errorcluster)  [unwired: 1 in, 1 out]
              }
              frame 7 {
                n138 = Fract/Exp String To Number(use system decimal point (T)=TRUE, string=w366) -> (number=w364:dbl)  [unwired: 2 in, 1 out]
                n139 = To Variant(anything=w364) -> (Variant=w365:variant)
                n140 = property class="Ctl"(reference=w367, "Value"=w365) -> (error out=w368:errorcluster)  [unwired: 1 in, 1 out]
              }
              frame 8 {
                n141 = Fract/Exp String To Number(use system decimal point (T)=TRUE, string=w372) -> (number=w370:dbl)  [unwired: 2 in, 1 out]
                n142 = To Variant(anything=w370) -> (Variant=w371:variant)
                n143 = property class="Ctl"(reference=w373, "Value"=w371) -> (error out=w374:errorcluster)  [unwired: 1 in, 1 out]
              }
            }
          }
        }
        frame Error {
          n144 = call <vilib>:"Clear Errors.vi"("error in (no error)"=w377, "specific error code to clear (0: all)"=4) -> ("error out"=w376:errorcluster)  [unwired: 4 in, 1 out]
        }
      }
      n145 = case shown="No Error" w286 {
        selector: w286 -> [w393 w512]
        tunnel: w291 -> [w394 w513]
        tunnel: [w381 w512] -> w290
        tunnel: [w392 w513] -> w289
        tunnel: [w385 -1.0] -> w285
        tunnel: w279 -> [w384 _]
        tunnel: w278 -> [w378 _]
        frame No Error {
          n146 = while {
            tunnel: w394 -> [w510]
            tunnel: w393 -> [w509]
            tunnel: [w510] -> w389
            tunnel: [w509] -> w391
            tunnel: [w495] -> w380
            stop <- "Close 2" stop-if-true
            # "Main Loop"
            n147 = Unbundle By Name("T2E2") -> ("Vmax (V)"=w506:dbl, "Vmin (V)"=w505:dbl, "Taxa de Aquisição (Hz)"=w504:dbl, "Resolução (bits)"=w503:dbl, "Amplificação (V/V)"=w502:dbl, "V+(V)"=w501:dbl, "V- (V)"=w500:dbl, "LSB (V)"=w499:dbl)
            n148 = Build Array(w506, w505, w504, w503, w502, w501, w500, w499) -> (w494:dbl[])
            n149 = case shown="True" "Help? 3" {
              frame False {
              }
              frame True {
                n150 = call "Greteer.vi"() -> ()  [unwired: 10 in, 2 out]
              }
            }
            n151 = Number To Fractional String(use system decimal point (T)=TRUE, number=w494, width (-)=i16 5, precision (6)=i16 12) -> (F-format string=w495:string[])
          }
          n152 = Set File Size(4:w391, 6:i64 0 ("size (in bytes)"), 7:w389) -> (0:w390:errorcluster, 3:w388:refnum<file>)
          n153 = Array Size(array=w384) -> (size(s)=w383:i32)
          n154 = call "logfile.vi"("Locale"="tut2ex2" ("from"), "Text In"=w380, "Path In"=w378) -> ()  [unwired: 7 in, 2 out]
          n155 = Write to Text File(file (use dialog)=w388, text=w380, error in=w390) -> (refnum out=w392:refnum<file>, error out=w382:errorcluster)  [unwired: 1 in, 1 out]
          n156 = for {
            shift-right: [w401] -> w386
            shift-left: _ -> [w400]
            tunnel: w384 -> [w398] mode=indexing
            tunnel: w382 -> [w397]
            tunnel: [w395] -> w381
            i -> [w402]
            n157 = Increment(x=w402) -> (x+1=w399:i32)
            n158 = case shown="8" w399 {
              tunnel: [0 ("f") w413 w424 w435 w446 w457 w468 w479 w490] -> w396
              tunnel: w398 -> [_ w410 w421 w432 w443 w454 w465 w476 w487]
              tunnel: w397 -> [_ w409 w420 w431 w442 w453 w464 w475 w486]
              tunnel: [errorcluster {"status"=FALSE, "code"=0, "source"=""} ("error out") w407 w418 w429 w440 w451 w462 w473 w484] -> w395
              frame 0, Default {
              }
              frame 1 {
                n159 = property class="Ctl"(reference=w410, error in=w409) -> (error out=w408:errorcluster, "Value"=w411:variant)  [unwired: 1 out]
                n160 = Variant To Data(error in=w408, type=0.0 ("y"), Variant=w411) -> (data=w405:dbl, error out=w407:errorcluster)
                n161 = Not Equal To 0?(x=w405) -> (x != 0?=w406:bool)
                n162 = Select(t=1, s=w406, f=0) -> (s? t:f=w413:i32)
              }
              frame 2 {
                n163 = property class="Ctl"(reference=w421, error in=w420) -> (error out=w419:errorcluster, "Value"=w422:variant)  [unwired: 1 out]
                n164 = Variant To Data(error in=w419, type=0.0 ("y"), Variant=w422) -> (data=w416:dbl, error out=w418:errorcluster)
                n165 = Not Equal To 0?(x=w416) -> (x != 0?=w417:bool)
                n166 = Select(t=1, s=w417, f=0) -> (s? t:f=w424:i32)
              }
              frame 3 {
                n167 = property class="Ctl"(reference=w432, error in=w431) -> (error out=w430:errorcluster, "Value"=w433:variant)  [unwired: 1 out]
                n168 = Variant To Data(error in=w430, type=0.0 ("y"), Variant=w433) -> (data=w427:dbl, error out=w429:errorcluster)
                n169 = Not Equal To 0?(x=w427) -> (x != 0?=w428:bool)
                n170 = Select(t=1, s=w428, f=0) -> (s? t:f=w435:i32)
              }
              frame 4 {
                n171 = property class="Ctl"(reference=w443, error in=w442) -> (error out=w441:errorcluster, "Value"=w444:variant)  [unwired: 1 out]
                n172 = Variant To Data(error in=w441, type=0.0 ("y"), Variant=w444) -> (data=w438:dbl, error out=w440:errorcluster)
                n173 = Not Equal To 0?(x=w438) -> (x != 0?=w439:bool)
                n174 = Select(t=1, s=w439, f=0) -> (s? t:f=w446:i32)
              }
              frame 5 {
                n175 = property class="Ctl"(reference=w454, error in=w453) -> (error out=w452:errorcluster, "Value"=w455:variant)  [unwired: 1 out]
                n176 = Variant To Data(error in=w452, type=0.0 ("y"), Variant=w455) -> (data=w449:dbl, error out=w451:errorcluster)
                n177 = Not Equal To 0?(x=w449) -> (x != 0?=w450:bool)
                n178 = Select(t=1, s=w450, f=0) -> (s? t:f=w457:i32)
              }
              frame 6 {
                n179 = property class="Ctl"(reference=w465, error in=w464) -> (error out=w463:errorcluster, "Value"=w466:variant)  [unwired: 1 out]
                n180 = Variant To Data(error in=w463, type=0.0 ("y"), Variant=w466) -> (data=w460:dbl, error out=w462:errorcluster)
                n181 = Not Equal To 0?(x=w460) -> (x != 0?=w461:bool)
                n182 = Select(t=1, s=w461, f=0) -> (s? t:f=w468:i32)
              }
              frame 7 {
                n183 = property class="Ctl"(reference=w476, error in=w475) -> (error out=w474:errorcluster, "Value"=w477:variant)  [unwired: 1 out]
                n184 = Variant To Data(error in=w474, type=0.0 ("y"), Variant=w477) -> (data=w471:dbl, error out=w473:errorcluster)
                n185 = Not Equal To 0?(x=w471) -> (x != 0?=w472:bool)
                n186 = Select(t=1, s=w472, f=0) -> (s? t:f=w479:i32)
              }
              frame 8 {
                n187 = property class="Ctl"(reference=w487, error in=w486) -> (error out=w485:errorcluster, "Value"=w488:variant)  [unwired: 1 out]
                n188 = Variant To Data(error in=w485, type=0.0 ("y"), Variant=w488) -> (data=w482:dbl, error out=w484:errorcluster)
                n189 = Not Equal To 0?(x=w482) -> (x != 0?=w483:bool)
                n190 = Select(t=1, s=w483, f=0) -> (s? t:f=w490:i32)
              }
            }
            n191 = Add(x=w396, y=w400) -> (x+y=w401:i32)
          }
          n192 = Divide(x=w386, y=w383) -> (x/y=w385:dbl)
        }
        frame Error {
        }
      }
    }
    frame "0" {
      n193 = control-ref of="TEVAL"() -> (w516:refnum<vi>)
      n194 = property class="Clust (strict)"(reference=w516) -> ("Controls[]"=w518:refnum<vi>[])  [unwired: 1 in, 2 out]
      n195 = Build Path(base path=w514, name or relative path="teval.txt") -> (appended path=w532:path)
      n196 = Open/Create/Replace File(file path (use dialog)=w532, error in=w531, operation (0:open)=T9."open or create", access (0:read/write)=enum16{"read/write", "read-only", "write-only"}."read/write") -> (refnum out=w528:refnum<file>, error out=w527:errorcluster)  [unwired: 2 in, 1 out]
      n197 = Array Size(array=w518) -> (size(s)=w519:i32)
      n198 = Read from Text File(file (use dialog)=w528, count=w519, error in=w527) -> (refnum out=w526:refnum<file>, text=w522:string[], error out=w523:errorcluster)  [unwired: 1 in, 1 out]
      n199 = case shown="No Error" w523 {
        selector: w523 -> [w536 w578]
        tunnel: w522 -> [w537 _]
        tunnel: [w535 w577] -> w521
        tunnel: w518 -> [w534 _]
        frame No Error {
          n200 = for {
            tunnel: w537 -> [w547] mode=indexing
            tunnel: [w546] -> w535
            tunnel: w536 -> [w545]
            tunnel: w534 -> [w544] mode=indexing
            # "Initializer Loop"
            n201 = Scan From String(format string="%d", input string=w547, error in=w545) -> (error out=w542:errorcluster, output 1=w540:i32)  [unwired: 2 in, 2 out]
            n202 = To Unsigned Long Integer(number=w540) -> (unsigned 32bit integer=w541:u32)
            n203 = case shown="No Error" w542 {
              selector: w542 -> [w549 w574]
              tunnel: w541 -> [w551 _]
              tunnel: [w550 radiobutton010."2" ("Radio Buttons")] -> w539
              tunnel: [w548 w574] -> w538
              frame No Error {
                n204 = case shown="10" w551 {
                  tunnel: [radiobutton010."No Selection" ("Radio Buttons") radiobutton010."1" ("Radio Buttons") radiobutton010."2" ("Radio Buttons") radiobutton010."3" ("Radio Buttons") radiobutton010."4" ("Radio Buttons") radiobutton010."5" ("Radio Buttons") radiobutton010."6" ("Radio Buttons") radiobutton010."7" ("Radio Buttons") radiobutton010."8" ("Radio Buttons") radiobutton010."9" ("Radio Buttons") radiobutton010."10" ("Radio Buttons")] -> w550
                  tunnel: w549 -> [w552 w555 w557 w559 w561 w563 w565 w567 w569 w571 w573]
                  tunnel: [w552 w555 w557 w559 w561 w563 w565 w567 w569 w571 w573] -> w548
                  frame 0, Default {
                  }
                  frame 1 {
                  }
                  frame 2 {
                  }
                  frame 3 {
                  }
                  frame 4 {
                  }
                  frame 5 {
                  }
                  frame 6 {
                  }
                  frame 7 {
                  }
                  frame 8 {
                  }
                  frame 9 {
                  }
                  frame 10 {
                  }
                }
              }
              frame Error {
              }
            }
            n205 = property class="Ctl"(reference=w544, error in=w538, "Val(Sgnl)"=w539) -> (error out=w546:errorcluster)  [unwired: 1 out]
          }
        }
        frame Error {
          n206 = call <vilib>:"Clear Errors.vi"("error in (no error)"=w578, "specific error code to clear (0: all)"=4) -> ("error out"=w577:errorcluster)  [unwired: 4 in, 1 out]
        }
      }
      n207 = case shown="No Error" w521 {
        selector: w521 -> [w594 w627]
        tunnel: w526 -> [w595 w628]
        tunnel: [w582 w627] -> w525
        tunnel: [w593 w628] -> w524
        tunnel: [w586 -1.0] -> w520
        tunnel: w518 -> [w585 _]
        tunnel: w514 -> [w579 _]
        frame No Error {
          n208 = while {
            tunnel: w595 -> [w625]
            tunnel: w594 -> [w624]
            tunnel: [w625] -> w590
            tunnel: [w624] -> w592
            tunnel: [w611] -> w581
            stop <- "Close 3" stop-if-true
            # "Main Loop"
            n209 = Unbundle By Name("TEVAL") -> ("Tamanho"=w623:T11, "Tempo Utilizado"=w622:T11, "Conteúdo Adequado"=w621:T11, "Conteúdo Claro / Coeso"=w620:T11, "Adequação à proposta de Reforço das Aulas de Laboratório e de Ensino de LabVIEW"=w619:T11, "Contexto dos Problemas Sugeridos"=w618:T11, "Contexto das Ferramentas Apresentadas"=w617:T11, "Ajuda na compreensão de outras matérias"=w616:T11, "compreensão de programação em LabVIEW"=w615:T11, "compreensão da teoria apresentada"=w614:T11)
            n210 = Build Array(w623, w622, w621, w620, w619, w618, w617, w616, w615, w614) -> (w613:T12)
            n211 = Number To Decimal String(number=w613, width (-)=i16 2) -> (decimal integer string=w611:string[])
          }
          n212 = Set File Size(4:w592, 6:i64 0 ("size (in bytes)"), 7:w590) -> (0:w591:errorcluster, 3:w589:refnum<file>)
          n213 = call "logfile.vi"("Locale"="tut2eval" ("from"), "Text In"=w581, "Path In"=w579) -> ()  [unwired: 7 in, 2 out]
          n214 = Write to Text File(file (use dialog)=w589, text=w581, error in=w591) -> (refnum out=w593:refnum<file>, error out=w583:errorcluster)  [unwired: 1 in, 1 out]
          n215 = for {
            shift-right: [w607] -> w587
            shift-left: _ -> [w606]
            tunnel: w585 -> [w605] mode=indexing
            tunnel: w583 -> [w604]
            tunnel: [w603] -> w582
            w598 = radiobutton010."No Selection" ("y")
            # "Check for Valid Response"
            n216 = property class="Ctl"(reference=w605, error in=w604) -> (error out=w596:errorcluster, "Value"=w599:variant)  [unwired: 1 out]
            n217 = Variant To Data(error in=w596, type=w598, Variant=w599) -> (data=w597:T10, error out=w603:errorcluster)
            n218 = Not Equal?(x=w597, y=w598) -> (x != y?=w602:bool)
            n219 = Select(t=1, s=w602, f=0) -> (s? t:f=w608:i32)
            n220 = Add(x=w608, y=w606) -> (x+y=w607:i32)
          }
          n221 = Array Size(array=w585) -> (size(s)=w584:i32)
          n222 = Divide(x=w587, y=w584) -> (x/y=w586:dbl)
        }
        frame Error {
        }
      }
    }
  }
  "path" <- w18
  "Waveform Out" <- w13
  n223 = Build Array("Init tut2ex1") -> (w4:string[])
  n224 = call "logfile.vi"("Error In"=w2, "Locale"="tut2ex1", "Text In"=w4) -> ()  [unwired: 7 in, 2 out]
  n225 = flat-sequence {
    tunnel: w28 -> [w646]
    tunnel: w27 -> [w645]
    tunnel: [w629] -> w21
    tunnel: [w642] -> w20
    tunnel: w19 -> [w642]
    tunnel: w11 -> [w639]
    tunnel: ["Respostas salvas com sucesso!" ("message")] -> w10
    tunnel: w9 -> [w634]
    frame #0 {
      w644 = TRUE ("Front Panel Window:Show Menu Bar")
      n226 = Close File(refnum=w645, error in=w646) -> (error out=w643:errorcluster)  [unwired: 1 out]
      n227 = control-ref of="This VI"() -> (w641:refnum<vi>)
      n228 = property class="VI"(reference=w641, error in=w643, "Front Panel.ShowMenuBar"=w644, "TB.Visible"=w644) -> (reference out=w632:refnum<vi>, error out=w631:errorcluster)
      n229 = Build Path(base path=w639, name or relative path="moodle_files") -> (appended path=w636:path)
      n230 = Build Path(base path=w636, name or relative path=w634) -> (appended path=w635:path)
      n231 = invoke class="VI" method="FP.Get Image"(reference=w632, error in=w631, "visible area only"=FALSE ("Visible Area Only")) -> (error out=w630:errorcluster, "image data"=w640:T13)  [unwired: 3 in, 4 out]
      n232 = call <vilib>:"Write PNG File.vi"("error in (no error)"=w630, "image data"=w640, "path to PNG file"=w635) -> ("error out"=w629:errorcluster)  [unwired: 7 in, 1 out]
    }
  }
  n233 = One Button Dialog(message=w10) -> ()  [unwired: 1 in, 1 out]
  "error out" <- w21
  "Done" <- w20
